vi "LOGIC_ccd_setup_image.vi"(6 "raw bpp":i32=16, 7 "log_file":path, 8 "error in (no error)":errorcluster, 11 "Database RefNum in":T1) -> (0 "error out":errorcluster, 1 "usc_tmout":i32, 2 "orig name":string)   [LabVIEW 2016]
uses:
  DBSHAND/private/vis/DatabaseHand_RefNum.ctl
  DBSHAND/private/vis/DatabaseHand_Element_Get(I32).vi
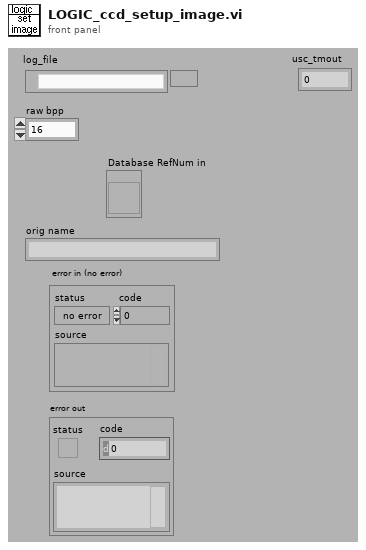
[diagram p1: front panel]
types:
  T1 = typedef "DatabaseHand_RefNum.ctl" = refnum<vi>
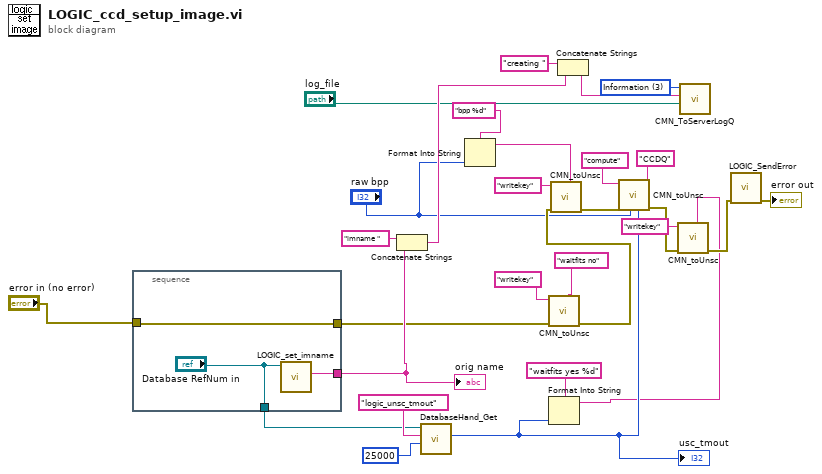
[diagram p0: block diagram]
diagram:
  w22 = u16 3 items=["command", "imediateReply", "Callback Reply", "Information"] ("type")
  n1 = stacked-sequence {
    tunnel: [w32] -> w17
    tunnel: ["Database RefNum in"] -> w10
    tunnel: "error in (no error)" -> [w30]
    tunnel: [w30] -> w7
    frame #0 {
      n2 = call "LOGIC_set_imname.vi"("Database RefNum in"="Database RefNum in") -> ("imname"=w32:string)  [unwired: 10 out]
    }
  }
  "orig name" <- w17
  n3 = Concatenate Strings("imname " ("Substring"), w17) -> (w20:string)
  n4 = call-poly "DatabaseHand_Get.vi"("default value"=25000, "name"="logic_unsc_tmout", "Database RefNum in"=w10) -> ("value"=w8:i32)  [unwired: 2 in, 6 out]
  "usc_tmout" <- w8
  n5 = Format Into String(format string="bpp %d" ("key"), "raw bpp") -> (resulting string=w14:string)  [unwired: 2 in, 1 out]
  n6 = call "CMN_toUnsc.vi"("key"="waitfits no", "error in (no error)"=w7, "command"="writekey") -> ("error out"=w23:errorcluster)  [unwired: 6 in, 2 out]
  n7 = Format Into String(format string="waitfits yes %d" ("key"), w8) -> (resulting string=w3:string)  [unwired: 2 in, 1 out]
  n8 = call "CMN_toUnsc.vi"("key"=w14, "error in (no error)"=w23, "command"="writekey") -> ("error out"=w28:errorcluster)  [unwired: 6 in, 2 out]
  n9 = Concatenate Strings("creating " ("string"), w20) -> (w19:string)
  n10 = call "CMN_toUnsc.vi"("responseQ"="CCDQ", "ms timeout (-1)"=w8, "bpp"="raw bpp", "error in (no error)"=w28, "command"="compute") -> ("error out"=w5:errorcluster)  [unwired: 4 in, 2 out]
  n11 = call "CMN_toUnsc.vi"("key"=w3, "error in (no error)"=w5, "command"="writekey") -> ("error out"=w4:errorcluster)  [unwired: 6 in, 2 out]
  n12 = call "CMN_ToServerLogQ.vi"("file"="log_file", "string"=w19, "type"=w22) -> ()  [unwired: 3 in, 5 out]
  n13 = call "LOGIC_SendError.vi"("error in (no error)"=w4) -> ("error out"=→"error out":errorcluster)  [unwired: 2 in, 8 out]
